vi "Engine-Event-WindowDisplayChanged.vi"(8 "error in (no error)":errorcluster, 9 "Display ID":T1, 10 "Timestamp":u64, 11 "GLF Window in":refnum<class "Window.lvclass">) -> (0 "error out":errorcluster, 3 "GLF Window out":refnum<class "Window.lvclass">)   [LabVIEW 2020, in "GLF.lvlib" / "Window.lvclass"]
uses:
  Window.lvclass
  Window.lvclass/Window.ctl
  WindowEventInterface/WindowEventInterface.lvclass
  <vilib>/Saukko/LV SDL3/Sources/SDL3/Video/DisplayID--integer.ctl
  <vilib>/Saukko/LV SDL3/Sources/SDL3/Video/Video.lvlib
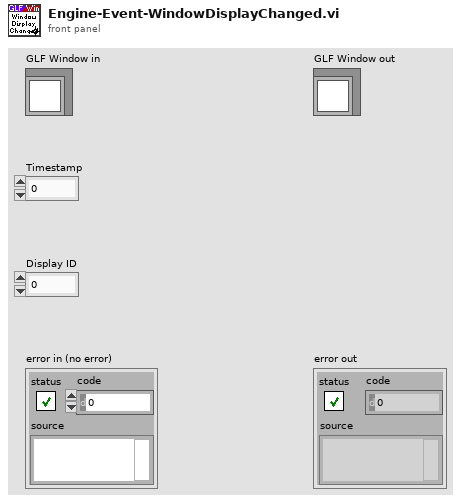
[diagram p1: front panel]
types:
  T1 = typedef "SDL3.lvlib/Video.lvlib/DisplayID--integer.ctl" = u32
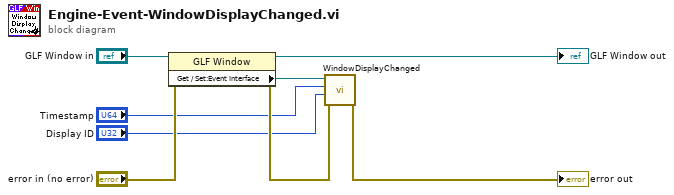
[diagram p0: block diagram]
diagram:
  n1 = property class="GLF Window"(reference="GLF Window in", error in="error in (no error)") -> (reference out=→"GLF Window out":refnum<class "Window.lvclass">, error out=w4:errorcluster, "Get / Set:Event Interface"=w5:refnum<class "WindowEventInterface.lvclass">)
  n2 = call-dynamic "WindowDisplayChanged.vi"("error in (no error)"=w4, "DisplayID"="Display ID", "Timestamp"="Timestamp", "WindowEventInterface in"=w5) -> ("error out"=→"error out":errorcluster)  [unwired: 7 in]
